vi "SetListData.vi"(4 "error in (no error)":errorcluster, 5 "Value":T1(array[cluster])=[{"Tag"="1", "Name"="1", "Symbol"=0, "Checked"=FALSE, "ParentTag"="t"}], 6 "Container State":T3, 7 "Display State In":T2={"Items"=[{"Tag"="1", "Name"="1", "Symbol"=0, "Checked"=FALSE, "ParentTag"="t"}], "CellHeight"=0}) -> (0 "error out":errorcluster, 3 "Display State Out":T2={"Items"=[{"Tag"="1", "Name"="1", "Symbol"=0, "Checked"=FALSE, "ParentTag"="t"}], "CellHeight"=0})   [LabVIEW 2020, in "XSubMenu.xctl"]
uses:
  XSubMenu.xctl
  <vilib>/_xctls/Container State.ctl
  XSubMenu-State.ctl
  <vilib>/_xctls/XControlSupport.lvlib
panel:
  # "Replace the Value Control below with a Control of desired type.\nDo not remove this Control or the others from the connector pane.\nDo not change the connector pane pattern.\nThe Value control should always be the third terminal from top on the input side in the connector pane."
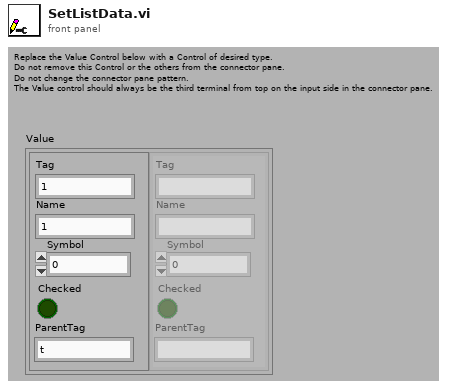
[diagram p1: front panel]
types:
  T1 = cluster{"Tag":string, "Name":string, "Symbol":i32, "Checked":bool, "ParentTag":string}[]
  T2 = typedef "XSubMenu.xctl/XSubMenu-State.ctl" = cluster{"Items":cluster{"Tag":string, "Name":string, "Symbol":i32, "Checked":bool, "ParentTag":string}[], "CellHeight":i32}
  T3 = typedef "XControlSupport.lvlib/Container State.ctl" = cluster{"Indicator?":bool, "Run Mode?":bool, " Refnum":refnum<vi>}
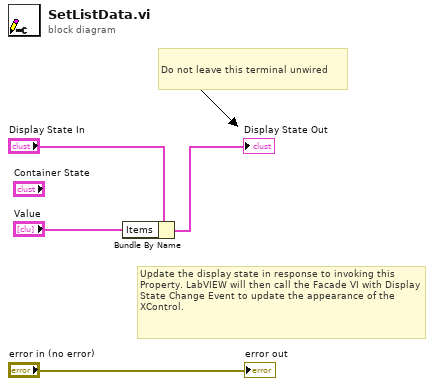
[diagram p0: block diagram]
diagram:
  # "Do not leave this terminal unwired"
  # "Update the display state in response to invoking this Property. LabVIEW will then call the Facade VI with Display State Change Event to update the appearance of the XControl."
  n1 = Bundle By Name(cluster="Display State In", "Items"="Value") -> (→"Display State Out":T2)
  "error out" <- "error in (no error)"
